vi "Connect.vi"(8 "error in":errorcluster, 11 "SL_SC in":refnum<class "SL_SC.lvclass">) -> (0 "error out":errorcluster, 3 "SL_SC out":refnum<class "SL_SC.lvclass">)   [LabVIEW 2019, in "SL_SC.lvlib" / "SL_SC.lvclass"]
doc: "This override VI is a carryover override from the parent class, children classes *must* override this VI and therefore the parent class must contain this VI to maintain the override rules."
uses:
  Library/SL_SC.lvclass
  C:/Users/Public/Documents/Development/builds/Instruments/Instruments.lvlibp/Library/Instruments.lvclass
  Library/SL_SC.lvclass/SL_SC.ctl
  builds/Instruments/Instruments.lvlibp/Accessors/Read Resource.vi
  <vilib>/SLSC/Initialize Session with Devices.vi
  builds/Instruments/DIG_IO.lvlibp/Library/DIG_IO.lvclass
  <vilib>/SLSC/SLSC.lvlib
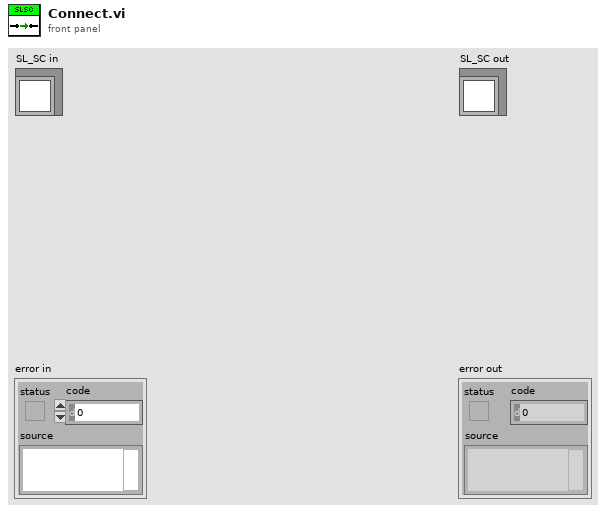
[diagram p1: front panel]
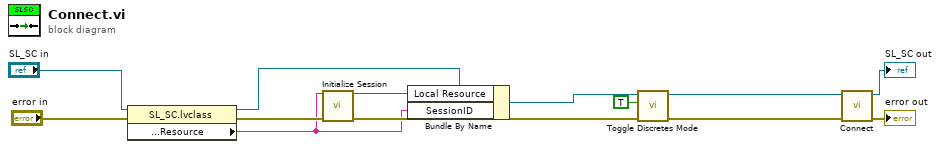
[diagram p0: block diagram]
diagram:
  n1 = property class="SL_SC.lvclass"(reference="SL_SC in", error in="error in") -> (reference out=w4:refnum<class "SL_SC.lvclass">, error out=w6:errorcluster, "Accessors:Configuration:Resource"=w1:string)
  n2 = call-poly <vilib>:"Initialize Session.vi"("devices"=w1, "error in (no error)"=w6) -> ("session out"=w3:refnum<k21>, "error out"=w8:errorcluster)  [unwired: 12 in]
  n3 = Bundle By Name(cluster=w4, "Local Resource"=w3, "SessionID"=w1) -> (w2:refnum<class "SL_SC.lvclass">)
  n4 = call "Toggle Discretes Mode.vi"("error in"=w8, "Discrete_Enable"=TRUE, "SL_SC in"=w2) -> ("error out"=w10:errorcluster, "SL_SC out"=w11:refnum<class "SL_SC.lvclass">)  [unwired: 7 in]
  n5 = call-parent "Connect.vi"("error in"=w10, "DIG_IO in"=w11) -> ("error out"=→"error out":errorcluster, "DIG_IO out"=→"SL_SC out":refnum<class "SL_SC.lvclass">)  [unwired: 8 in]
